vi "circularCounter32bit.vi"(7 "reset":bool, 9 "doStep":bool=TRUE, 11 "maxCount":u32) -> (0 "maxReached":bool, 2 "next":u32, 3 "index":u32)   [LabVIEW 2016]
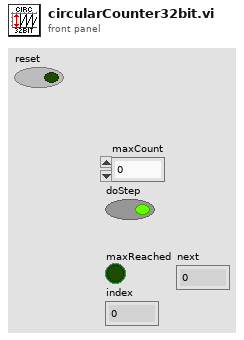
[diagram p1: front panel]
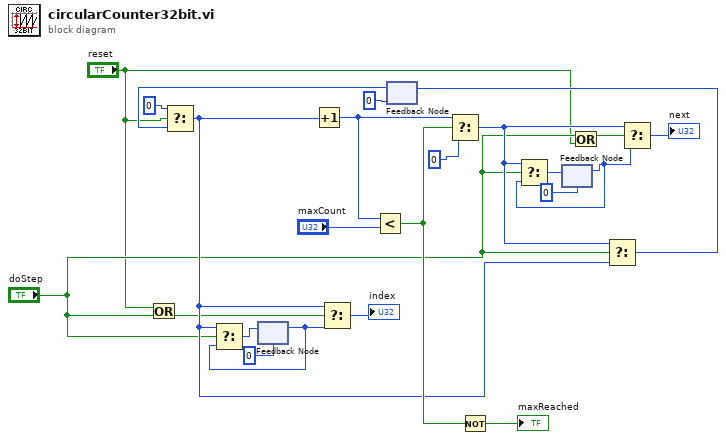
[diagram p0: block diagram]
diagram:
  n1 = Or(x="reset", y="doStep") -> (x .or. y?=w7:bool)
  n2 = feedback #1(u32 0 ("t")) -> (w14:u32)
  n3 = feedback #2(u32 0) -> (w21:u32)
  n4 = Select(t=u32 0, s="reset", f=w21) -> (s? t:f=w15:u32)
  n5 = Select(t=w15, s="doStep", f=w14) -> (s? t:f=w16:u32)
  n6 = feedback-in #1(w16) -> ()
  n7 = Increment(x=w15) -> (x+1=w22:u32)
  n8 = Select(t=w15, s=w7, f=w14) -> (s? t:f=→"index":u32)
  n9 = Less?(x=w22, y="maxCount") -> (x < y?=w20:bool)
  n10 = Select(t=w22, s=w20, f=u32 0) -> (s? t:f=w13:u32)
  n11 = Not(x=w20) -> (.not. x?=→"maxReached":bool)
  n12 = feedback #3(u32 0) -> (w11:u32)
  n13 = Select(t=w13, s="doStep", f=w11) -> (s? t:f=w12:u32)
  n14 = feedback-in #3(w12) -> ()
  n15 = Or(x="doStep", y="reset") -> (x .or. y?=w8:bool)
  n16 = Select(t=w13, s="doStep", f=w15) -> (s? t:f=w18:u32)
  n17 = feedback-in #2(w18) -> ()
  n18 = Select(t=w13, s=w8, f=w11) -> (s? t:f=→"next":u32)
